vi "RPC Get Test Paths and Version.vi"(5 "Test ID (\"\")":string, 8 "error in (no error)":errorcluster, 10 "Base Path (empty)":path, 11 "app reference (empty)":refnum<vi>) -> (0 "error out":errorcluster, 1 "Test Download component":path, 2 "Test Component Path":path, 3 "app reference":refnum<vi>, 4 "Version":cluster{"Version":string, "Build Number":u32})   [LabVIEW 2011]
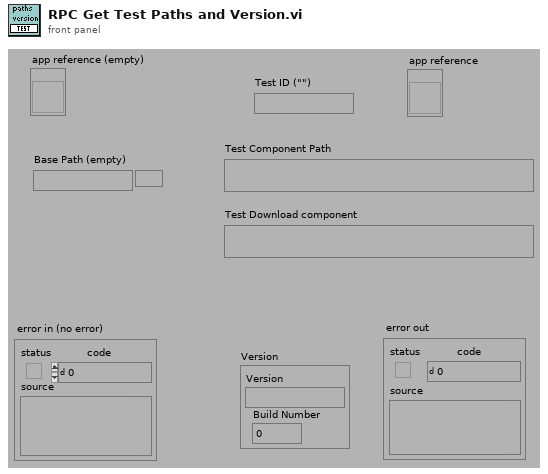
[diagram p1: front panel]
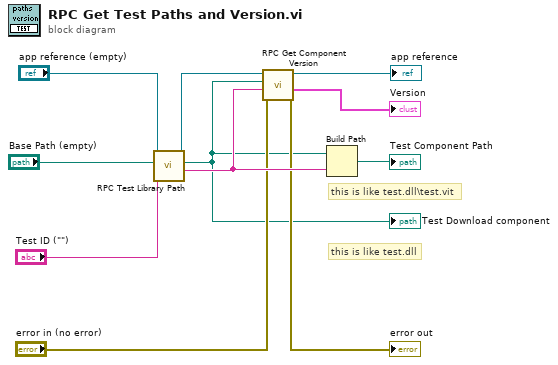
[diagram p0: block diagram]
diagram:
  # "this is like test.dll"
  # "this is like test.dll\\test.vit"
  n1 = call "RPC Test Library Path.vi"("Test ID (\"\")"="Test ID (\"\")", "Base Path (empty)"="Base Path (empty)", "App Ref (null: local)"="app reference (empty)") -> ("Component Name"=w9:string, "Library Path"=w1:path, "dup App Ref"=w2:refnum<vi>)  [unwired: 6 out]
  "Test Download component" <- w1
  n2 = call "RPC Get Component Version.vi"("error in (no error)"="error in (no error)", "Component (\"\")"=w9, "Component Library (empty)"=w1, "app reference (empty)"=w2) -> ("error out"=→"error out":errorcluster, "Component Version"=→"Version":cluster{"Version":string, "Build Number":u32}, "app reference"=→"app reference":refnum<vi>)  [unwired: 5 out]
  n3 = Build Path(base path=w1, name or relative path=w9) -> (appended path=→"Test Component Path":path)
